vi "DIO test.vi"() -> ()   [LabVIEW 2017]
uses:
  <vilib>/FPGAPlugInAG/PXI-7811R/niLvFpga_Open_PXI-7811R.vi
  <vilib>/rvi/interface/common/dynamic/niFpgaDynamicAddResources.vi
  <vilib>/Utility/error.llb/Error Cluster From Error Code.vi
  <vilib>/rvi/errors/niLvFpgaAdjustHostInterfaceError.vi
  <vilib>/FPGAPlugInAG/Dynamic/niLvFpga_Run_Dynamic.vi
  <vilib>/FPGAPlugInAG/Dynamic/niLvFpga_Reset_Dynamic.vi
  <vilib>/FPGAPlugInAG/Dynamic/niLvFpga_Abort_Dynamic.vi
  <vilib>/FPGAPlugInAG/Dynamic/niLvFpga_Close_Dynamic.vi
  <vilib>/rvi/interface/nirviOpenFPGA/nirviOpenFPGA.xnode
  FPGA Bitfiles/project1_FPGATarget_statemachine_2UlWpaN0YWU.lvbitx
  FPGA vi/state machine.vi
  <vilib>/rvi/interface/nirviMethod/nirviMethod.xnode
  <vilib>/rvi/interface/nirviReadWriteControl/nirviReadWriteControl.xnode
  <vilib>/rvi/interface/nirviCloseFPGA/nirviCloseFPGA.xnode
  <vilib>/rvi/errors/niLvFpgaMergeErrorWithErrorCode.vi
  <vilib>/FPGAPlugInAG/Dynamic/niLvFpga_WriteFifo_Dynamic.vi
  <vilib>/rvi/interface/Simulation/niFpgaSimulationCallBeginRW.vi
  NiFpgaLv.dll
panel:
  out "Boolean":bool=TRUE
  out "idle":bool
  out "real-time port D monitor":bool[](array[boolean])
  out "real-time port C monitor":bool[](array[boolean])
  out "real-time port B monitor":bool[](array[boolean])
  out "real-time port A monitor":bool[](array[boolean])
  out "run":bool
  out "reset":bool
  out "load":bool
  out "Numeric":i32
  out "error out":errorcluster
  in  "ouput 34":u64[](array[numeric])
  in  "ouput 12":u64[](array[numeric])
  in  "time":u64[](array[numeric])
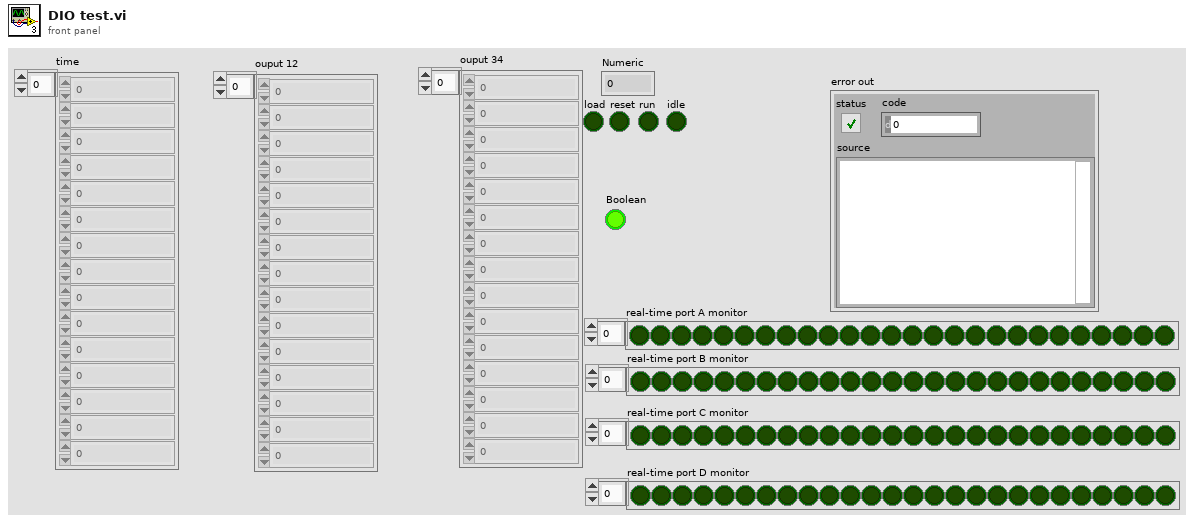
[diagram p1: front panel]
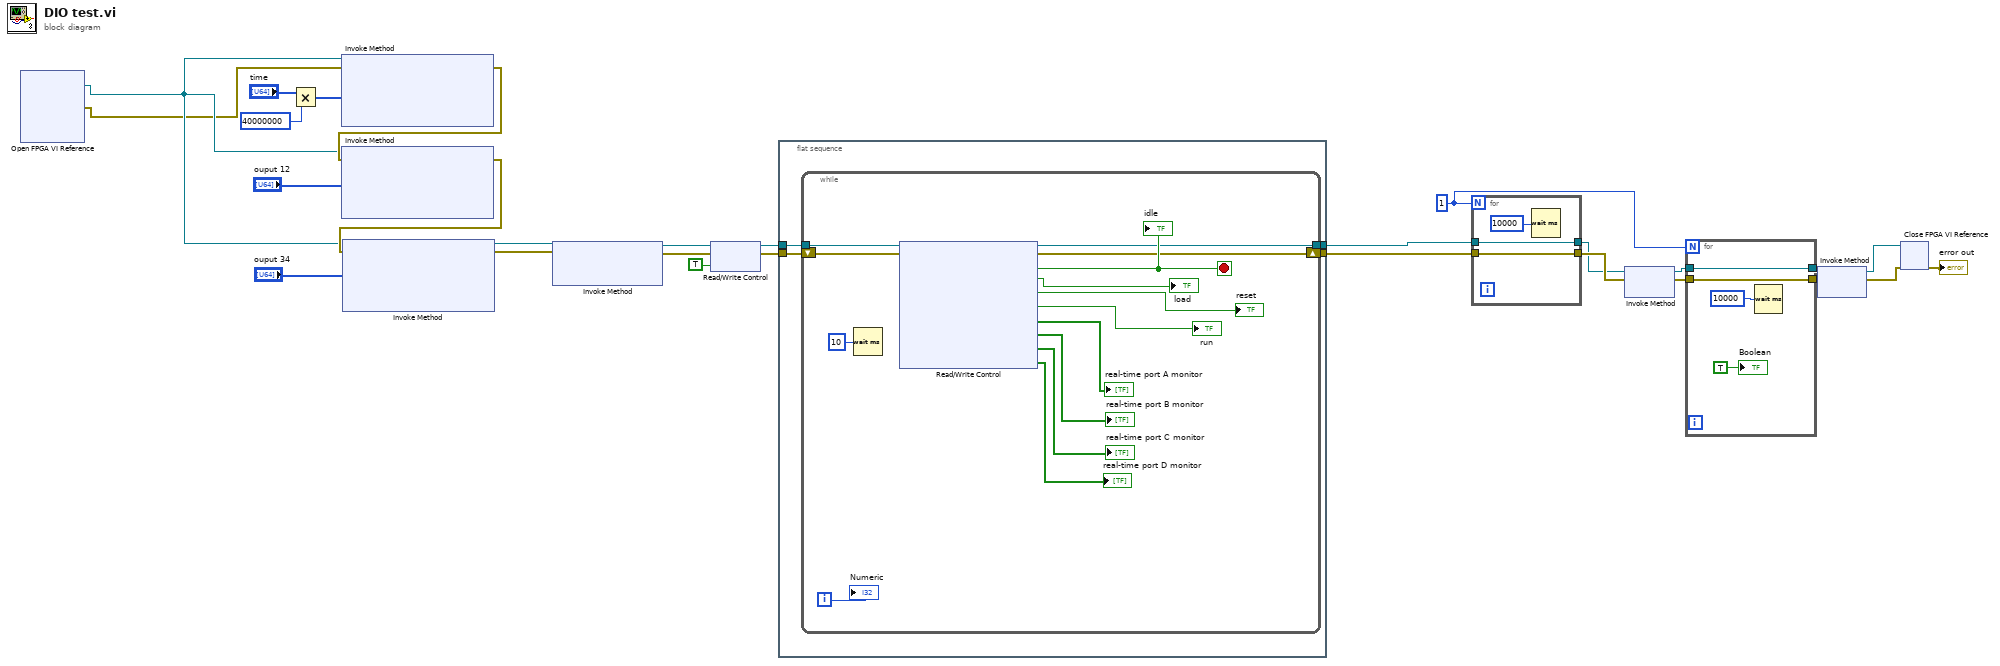
[diagram p0: block diagram]
diagram:
  w1 = 1
  n1 = xnode "Open FPGA VI Reference"() -> ("FPGA VI Reference Out"=w7:refnum<k20>, "error out"=w6:errorcluster)  [unwired: 2 in]
  n2 = Multiply(x="time", y=u64 40000000) -> (x*y=w16:u64[])
  n3 = xnode "Invoke Method"("FPGA VI Reference In"=w7, "error in"=w6, "Data"=w16) -> ("error out"=w26:errorcluster)  [unwired: 1 in, 2 out]
  n4 = xnode "Invoke Method"("FPGA VI Reference In"=w7, "error in"=w26, "Data"="ouput 12") -> ("error out"=w25:errorcluster)  [unwired: 1 in, 2 out]
  n5 = xnode "Invoke Method"("FPGA VI Reference In"=w7, "error in"=w25, "Data"="ouput 34") -> ("FPGA VI Reference Out"=w24:refnum<k20>, "error out"=w22:errorcluster)  [unwired: 1 in, 1 out]
  n6 = xnode "Invoke Method"("FPGA VI Reference In"=w24, "error in"=w22) -> ("FPGA VI Reference Out"=w23:refnum<k20>, "error out"=w21:errorcluster)  [unwired: 1 in]
  n7 = xnode "Read/Write Control"("FPGA VI Reference In"=w23, "error in"=w21, "Run"=TRUE) -> ("FPGA VI Reference Out"=w19:refnum<k20>, "error out"=w18:errorcluster)
  n8 = flat-sequence {
    tunnel: [w30] -> w11
    tunnel: [w29] -> w9
    tunnel: w19 -> [w32]
    tunnel: w18 -> [w31]
    frame #0 {
      n9 = while {
        tunnel: w32 -> [w46]
        shift-right: [w42] -> w30
        shift-left: w31 -> [w45]
        tunnel: [w41] -> w29
        i -> [w40]
        stop <- w43 stop-if-true
        n10 = Wait (ms)(milliseconds to wait=u32 10) -> ()  [unwired: 1 out]
        n11 = xnode "Read/Write Control"("FPGA VI Reference In"=w46, "error in"=w45) -> ("FPGA VI Reference Out"=w41:refnum<k20>, "error out"=w42:errorcluster, "idle LED"=w43:bool, "load LED"=→"load":bool, "reset LED"=→"reset":bool, "run LED"=→"run":bool, "real-time port A monitor"=→"real-time port A monitor":bool[], "real-time port B monitor"=→"real-time port B monitor":bool[], "real-time port C monitor"=→"real-time port C monitor":bool[], "real-time port D monitor"=→"real-time port D monitor":bool[])
        "idle" <- w43
        "Numeric" <- w40
      }
    }
  }
  n12 = for {
    N: w1 -> [_]
    tunnel: w11 -> [w49]
    tunnel: [w49] -> w10
    tunnel: w9 -> [w48]
    tunnel: [w48] -> w8
    n13 = Wait (ms)(milliseconds to wait=u32 10000) -> ()  [unwired: 1 out]
  }
  n14 = xnode "Invoke Method"("FPGA VI Reference In"=w8, "error in"=w10) -> ("FPGA VI Reference Out"=w5:refnum<k20>, "error out"=w4:errorcluster)
  n15 = for {
    N: w1 -> [_]
    tunnel: w4 -> [w53]
    tunnel: [w53] -> w2
    tunnel: w5 -> [w52]
    tunnel: [w52] -> w3
    n16 = Wait (ms)(milliseconds to wait=u32 10000) -> ()  [unwired: 1 out]
    "Boolean" <- TRUE
  }
  n17 = xnode "Invoke Method"("FPGA VI Reference In"=w3, "error in"=w2) -> ("FPGA VI Reference Out"=w12:refnum<k20>, "error out"=w13:errorcluster)
  n18 = xnode "Close FPGA VI Reference"("FPGA VI Reference In"=w12, "error in"=w13) -> ("error out"=→"error out":errorcluster)
